vi "Test.vi"   [LabVIEW 2020]
uses:
  Ctl/UpdateInsertableVICtl.ctl
  b95e2d39-9a72-4fb7-b733-c53d2ceefbbe.vi
  8616cbc6-d8ba-435f-9af2-03ccb79b2d5e.vi
  <userlib>/_NEVSTOP/Communicable State Machine(CSM)/_Polymophic/Build No-Reply Asynchronous Message with Arguments.vi
  <userlib>/_NEVSTOP/Communicable State Machine(CSM)/addons/API-String-Arugments-Support/_Support/Data To API String Arguments.vi
  <userlib>/_NEVSTOP/Communicable State Machine(CSM)/Communicable State Machine.lvlib
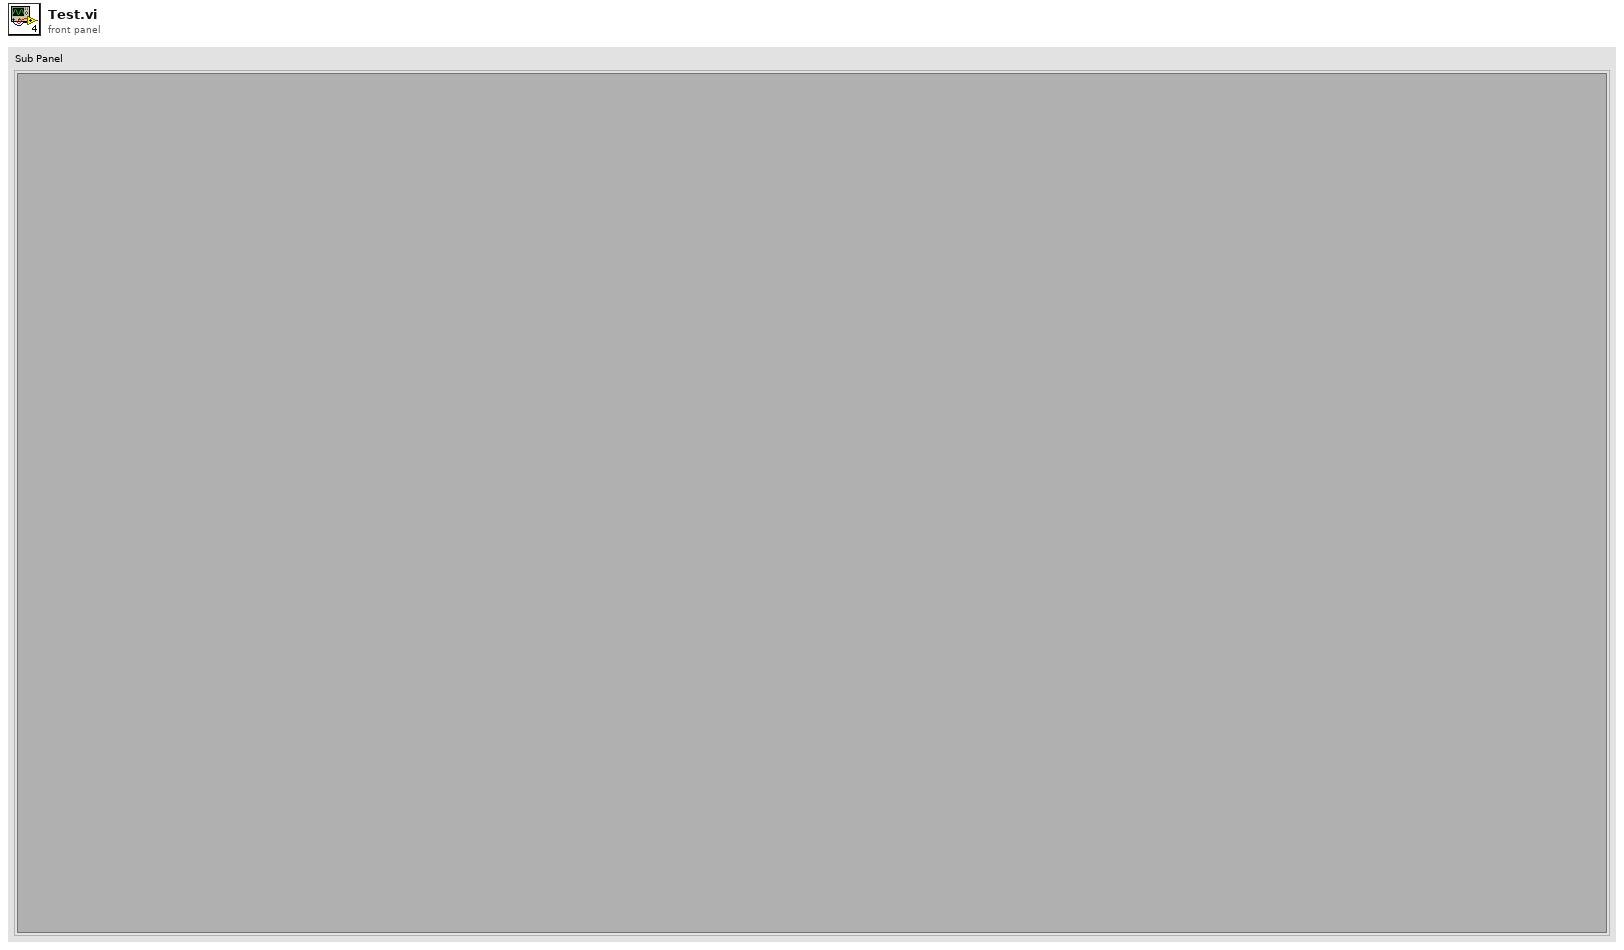
[diagram p1: front panel]
types:
  T1 = typedef "UpdateInsertableVICtl.ctl" = cluster{"Name":string, "VIPath":path}
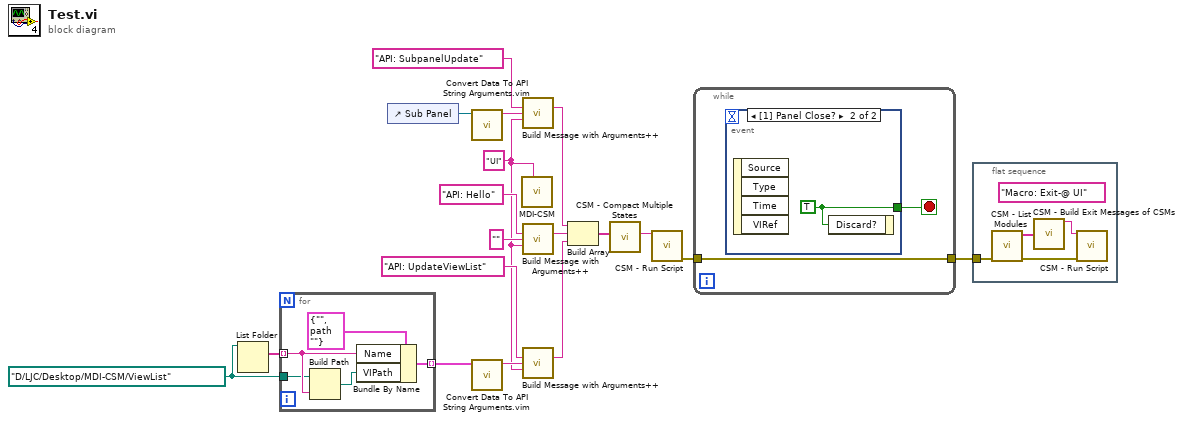
[diagram p0: block diagram]
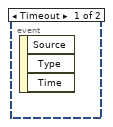
[diagram p2: hidden frame]
diagram:
  w7 = path "D:/LJC/Desktop/MDI-CSM/ViewList" ("path")
  w1 = "UI" ("Name (\"\" to Use UUID)")
  n1 = List Folder(path=w7) -> (filenames=w8:string[])  [unwired: 3 in, 3 out]
  n2 = for {
    tunnel: w8 -> [w22] mode=indexing
    tunnel: w7 -> [w21]
    tunnel: [w19] -> w6 mode=indexing
    n3 = Build Path(base path=w21, name or relative path=w22) -> (appended path=w20:path)
    n4 = Bundle By Name(cluster=T1 {"Name"="", "VIPath"=path ""} ("Array"), "Name"=w22, "VIPath"=w20) -> (w19:T1)
  }
  n5 = control-ref of="Sub Panel"() -> (w16:refnum<vi>)
  n6 = call "Convert Data To API String Arguments.vim"("Data"=w16) -> ("API String"=w15:string)  [unwired: 7 in, 1 out]
  n7 = call "Convert Data To API String Arguments.vim"("Data"=w6) -> ("API String"=w5:string)  [unwired: 7 in, 1 out]
  n8 = call "MDI-CSM.vi"("Name (\"\" to Use UUID)"=w1) -> ()  [unwired: 11 in]
  n9 = call-poly <userlib>:"Build Message with Arguments++.vi"("State With Arguments"="API: SubpanelUpdate", "Arguments (\"\")"=w15, "Target Module (\"\")"=w1) -> ("CSM Message String"=w14:string)  [unwired: 12 in]
  n10 = call-poly <userlib>:"Build Message with Arguments++.vi"("State With Arguments"="API: Hello", "Arguments (\"\")"="" ("Arguments (\"\")"), "Target Module (\"\")"=w1) -> ("CSM Message String"=w12:string)  [unwired: 12 in]
  n11 = call-poly <userlib>:"Build Message with Arguments++.vi"("State With Arguments"="API: UpdateViewList", "Arguments (\"\")"=w5, "Target Module (\"\")"=w1) -> ("CSM Message String"=w3:string)  [unwired: 12 in]
  n12 = Build Array(w14, w12, w3) -> (w11:string[])
  n13 = call <userlib>:"CSM - Compact Multiple States.vi"("Multiple States"=w11) -> ("States"=w10:string)  [unwired: 9 in]
  n14 = call <userlib>:"CSM - Run Script.vi"("CSM Scripts"=w10) -> ("error out"=w18:errorcluster)  [unwired: 12 in, 2 out]
  n15 = while {
    tunnel: w18 -> [w24]
    tunnel: [w24] -> w2
    stop <- w25 stop-if-true
    n16 = event shown="[1] Panel Close?" {
      selector: _ -> [_ _]
      dyn-events: _ -> [_ _]
      timeout: _ -> [_ _]
      tunnel: [_ w26] -> w25
      event Timeout {
        n17 = event-data() -> ()  [unwired: 1 in, 3 out]
      }
      event Panel Close? {
        w26 = TRUE ("Discard?")
        n18 = event-data() -> ()  [unwired: 1 in, 4 out]
        n19 = event-data("Discard?"=w26) -> ()  [unwired: 1 in, 1 out]
      }
    }
  }
  n20 = flat-sequence {
    tunnel: w2 -> [w29]
    frame #0 {
      (unwired) "Macro: Exit-@ UI" ("CSM Scripts")
      n21 = call <userlib>:"CSM - List Modules.vi"("Error In"=w29) -> ("error out"=w27:errorcluster, "Module Names"=w30:string[])  [unwired: 9 in]
      n22 = call <userlib>:"CSM - Build Exit Messages of CSMs.vi"("CSMs"=w30) -> ("States"=w28:string)  [unwired: 14 in]
      n23 = call <userlib>:"CSM - Run Script.vi"("CSM Scripts"=w28, "error in (no error)"=w27) -> ()  [unwired: 11 in, 3 out]
    }
  }
